vi "Begin.vi"() -> (0 "error out":errorcluster)   [LabVIEW 2023]
doc: "Called before other user functions, this VI is expected to open initial I/O refnums, load in file data, and do all program initialization. Notice that the <B>error out</B> terminal is simply used for data flow. Wiring it to other structures or subVIs ensures that this VI runs first."
uses:
  Robot Global Data.vi
  <vilib>/Rock Robotics/WPI/DriverStation/WPI_DriverStationRobotMode2.ctl
  <vilib>/Rock Robotics/WPI/Joystick/WPI_JoystickDeviceEnum.ctl
  <vilib>/Rock Robotics/WPI/ThirdParty/Phoenix-LabVIEW/Motor Controller/Controls/CTRE_Phoenix_MotorControl_FeedbackDevice_TalonFX.ctl
  <vilib>/Rock Robotics/WPI/ThirdParty/Phoenix-LabVIEW/Motor Controller/Controls/CTRE_Phoenix_MotorControl_NeutralMode.ctl
  <vilib>/Rock Robotics/WPI/ThirdParty/Phoenix-LabVIEW/Motor Controller/Controls/CTRE_Phoenix_MotorControl_TalonFXInvertType.ctl
  <vilib>/Rock Robotics/WPI/ThirdParty/Phoenix-LabVIEW/Motor Controller/Controls/CTRE_Phoenix_MotorControl_StatorCurrentLimitConfiguration.ctl
  <vilib>/Rock Robotics/WPI/ThirdParty/Phoenix-LabVIEW/CANCoder/Controls/CTRE_Phoenix_CANcoder_StatusFrame.ctl
  <vilib>/Rock Robotics/WPI/ThirdParty/REV Robotics/REVLib/Typedef/Spark MAX Idle Mode.ctl
  <vilib>/Rock Robotics/Network Tables/NT Write String Array.vi
  <vilib>/Rock Robotics/WPI/ThirdParty/Phoenix-LabVIEW/CANCoder/Controls/CTRE_Phoenix_CANcoder_SensorInitializationStrategy.ctl
  <vilib>/Rock Robotics/Network Tables/NT Write Number.vi
  <vilib>/Rock Robotics/Network Tables/NT Write String.vi
  <vilib>/Rock Robotics/WPI/ThirdParty/Phoenix-LabVIEW/CANdle/Controls/CTRE_Phoenix_CANdle_LEDStripType.ctl
  <vilib>/Rock Robotics/WPI/ThirdParty/Phoenix-LabVIEW/CANdle/Controls/CTRE_Phoenix_CANdle_Configurables.ctl
  <vilib>/Rock Robotics/SystemInterfaces/DIO/FPGA_DIOChannel.ctl
  <vilib>/Rock Robotics/Network Tables/NT Write Boolean.vi
  <vilib>/Rock Robotics/WPI/Switch/WPI_SwitchOpenLimit.vi
  <vilib>/Rock Robotics/WPI/ThirdParty/REV Robotics/REVLib/SubVI/Public/SPARK Open Brushless.vi
  <vilib>/Rock Robotics/WPI/ThirdParty/REV Robotics/REVLib/Typedef/Closed Loop Voltage Mode.ctl
  <vilib>/Rock Robotics/WPI/ThirdParty/REV Robotics/REVLib/Typedef/SPARK PID Gains.ctl
  <vilib>/Rock Robotics/WPI/ThirdParty/REV Robotics/REVLib/Typedef/SPARK Feedback Sensor.ctl
  <vilib>/Rock Robotics/WPI/ThirdParty/REV Robotics/REVLib/SubVI/Public/SPARK Configure Closed Loop Basic.vi
  <vilib>/Rock Robotics/WPI/ThirdParty/REV Robotics/REVLib/SubVI/Public/SPARK Configure Closed Loop MAXMotion.vi
  <vilib>/Rock Robotics/WPI/ThirdParty/REV Robotics/REVLib/SubVI/Public/SPARK Configure Basic Idle Mode.vi
  <vilib>/Rock Robotics/WPI/ThirdParty/REV Robotics/REVLib/SubVI/Public/SPARK Configure Power Smart Current Limit.vi
  <vilib>/Rock Robotics/WPI/ThirdParty/REV Robotics/REVLib/SubVI/Public/SPARK Configure Encoder Conversion Factors.vi
  <vilib>/Rock Robotics/WPI/ThirdParty/REV Robotics/REVLib/SubVI/Public/SPARK Configure Closed Loop Gains.vi
  <vilib>/Rock Robotics/WPI/ThirdParty/REV Robotics/REVLib/SubVI/Public/SPARK Configure Closed Loop Voltage Mode.vi
  <vilib>/Rock Robotics/Network Tables/NT Write Numeric Array.vi
  <vilib>/Rock Robotics/WPI/ThirdParty/REV Robotics/REVLib/SubVI/Public/SPARK Configure Soft Limit Reverse.vi
  <vilib>/Rock Robotics/WPI/ThirdParty/REV Robotics/REVLib/SubVI/Public/SPARK Configure Soft Limit Forward.vi
panel:
  in  "error in":errorcluster
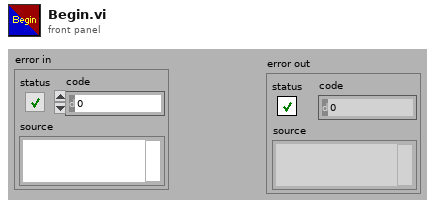
[diagram p1: front panel]
types:
  T1 = typedef "WPI_JoystickDeviceEnum.ctl" = enum16{"USB 0", "USB 1", "USB 2", "USB 3", "USB 4", "USB 5"}
  T2 = typedef "WPI_DriverStationRobotMode2.ctl" = enum16{"Autonomous Disabled", "Autonomous Enabled", "Teleop Disabled", "Teleop Enabled", "Disconnected", "Finish", "Test Disabled", "Test Enabled", "Emergency Stopped"}
  T3 = typedef "WPI_JoystickDevRef.ctl" = cluster{"Device":T1}
  T4 = typedef "CTRE_Phoenix_CANdle_Configurables.ctl" = cluster{"LED Strip Type":T5, "Brightness Scalar":dbl, "Disable LEDs when LoS":bool, "Status LED Off When Active":bool, "VBatOutputMode":u16}
  T5 = typedef "CTRE_Phoenix_CANdle_LEDStripType.ctl" = u16
  T6 = typedef "CTRE_Phoenix_CANdle_DeviceRef.ctl" = cluster{"DeviceStatus":errorcluster, "Device Number":u8, "Handle":u64, "UsageFrame":u32, "Library Path":path}
  T7 = typedef "SPARK Feedback Sensor.ctl" = enum16{"No Sensor", "Primary Encoder", "Analog Sensor", "Alternate or External Encoder", "Duty Cycle Sensor"}
  T8 = typedef "Spark MAX Idle Mode.ctl" = enum16{"Coast", "Brake"}
  T9 = typedef "SPARK PID Gains.ctl" = cluster{"kP":dbl, "kI":dbl, "kD":dbl}
  T10 = typedef "Closed Loop Voltage Mode.ctl" = enum16{"Disabled", "Voltage Output", "Voltage Compensation"}
  T11 = typedef "CTRE_Phoenix_MotorControl_StatorCurrentLimitConfiguration.ctl" = cluster{"Enable?":bool, "Current Limit":dbl, "Threshold Current":dbl, "Threshold Time":dbl}
  T12 = typedef "CTRE_Phoenix_MotorControl_NeutralMode.ctl" = enum8{"EEPROMSetting", "Override to Coast", "Override to Brake"}
  T13 = typedef "CTRE_Phoenix_MotorControl_TalonFXInvertType.ctl" = enum16{"Counter-Clockwise", "Clockwise"}
  T14 = typedef "FPGA_DIOChannel.ctl" = enum8{"DIO 0", "DIO 1", "DIO 2", "DIO 3", "DIO 4", "DIO 5", "DIO 6", "DIO 7", "DIO 8", "DIO 9", "DIO MXP 0", "DIO MXP 1", "DIO MXP 2", "DIO MXP 3", "DIO MXP 4", "DIO MXP 5", "DIO MXP 6", "DIO MXP 7", "DIO MXP 8", "DIO MXP 9", "DIO MXP 10", "DIO MXP 11", "DIO MXP 12", "DIO MXP 13", "DIO MXP 14", "DIO MXP 15", "SPI Port CS1", "SPI Port CS2", "SPI Port CS3", "SPI Port MISO", "SPI Port MOSI", "Invalid"}
  T15 = typedef "CTRE_Phoenix_CANcoder_SensorInitializationStrategy.ctl" = enum16{"Boot To Zero", "Boot To Absolute Position"}
  T16 = typedef "CTRE_Phoenix_MotorControl_FeedbackDevice_TalonFX.ctl" = i8
  T17 = typedef "CTRE_Phoenix_CANcoder_StatusFrame.ctl" = u32
  T18 = typedef "WPI_MotorControlDeviceRef.ctl" = cluster{"DeviceStatus":errorcluster, "Type":T19, "PWM":cluster{"PWM Channel":T20, "DeadBand":T21}, "CAN":cluster{"Device Number":u8, "SetOutput VI Ref":variant, "GetOutput VI Ref":variant, "Enable VI Ref":variant, "Disable VI Ref":variant, "Data":variant}, "Invert":bool, "DIO PWM":cluster{"PWM \"Enable\" Channel":T20, "DIOChannel":T14, "PWM Rate":dbl}}
  T19 = typedef "WPI_MotorControlType.ctl" = enum16{"PWM", "CAN", "DIO PWM"}
  T20 = typedef "FPGA_DIOPWMChannel.ctl" = enum8{"PWM 0", "PWM 1", "PWM 2", "PWM 3", "PWM 4", "PWM 5", "PWM 6", "PWM 7", "PWM 8", "PWM 9", "PWM MXP 0", "PWM MXP 1", "PWM MXP 2", "PWM MXP 3", "PWM MXP 4", "PWM MXP 5", "PWM MXP 6", "PWM MXP 7", "PWM MXP 8", "PWM MXP 9", "Invalid"}
  T21 = typedef "WPI_PWMDeadband.ctl" = cluster{"Name":string, "maxPositivePwm":i32, "minPositivePwm":i32, "centerPwm":i32, "maxNegativePwm":i32, "minNegativePwm":i32, "angularRange":u16}
  T22 = typedef "WPI_SwitchDevRef.ctl" = cluster{"DevStatus":errorcluster, "DIO Channel":T14, "CntIndex":T23, "Normally Closed":bool}
  T23 = typedef "FPGA_CounterCtrSystemIndex.ctl" = enum8{"Ctr 0", "Ctr 1", "Ctr 2", "Ctr 3", "Ctr 4", "Ctr 5", "Ctr 6", "Ctr 7", "Invalid"}
  T24 = typedef "CTRE_Phoenix_CANcoder_DeviceRef.ctl" = cluster{"DeviceStatus":errorcluster, "Device Number":u8, "Handle":u64, "UsageFrame":u32, "Library Path":path}
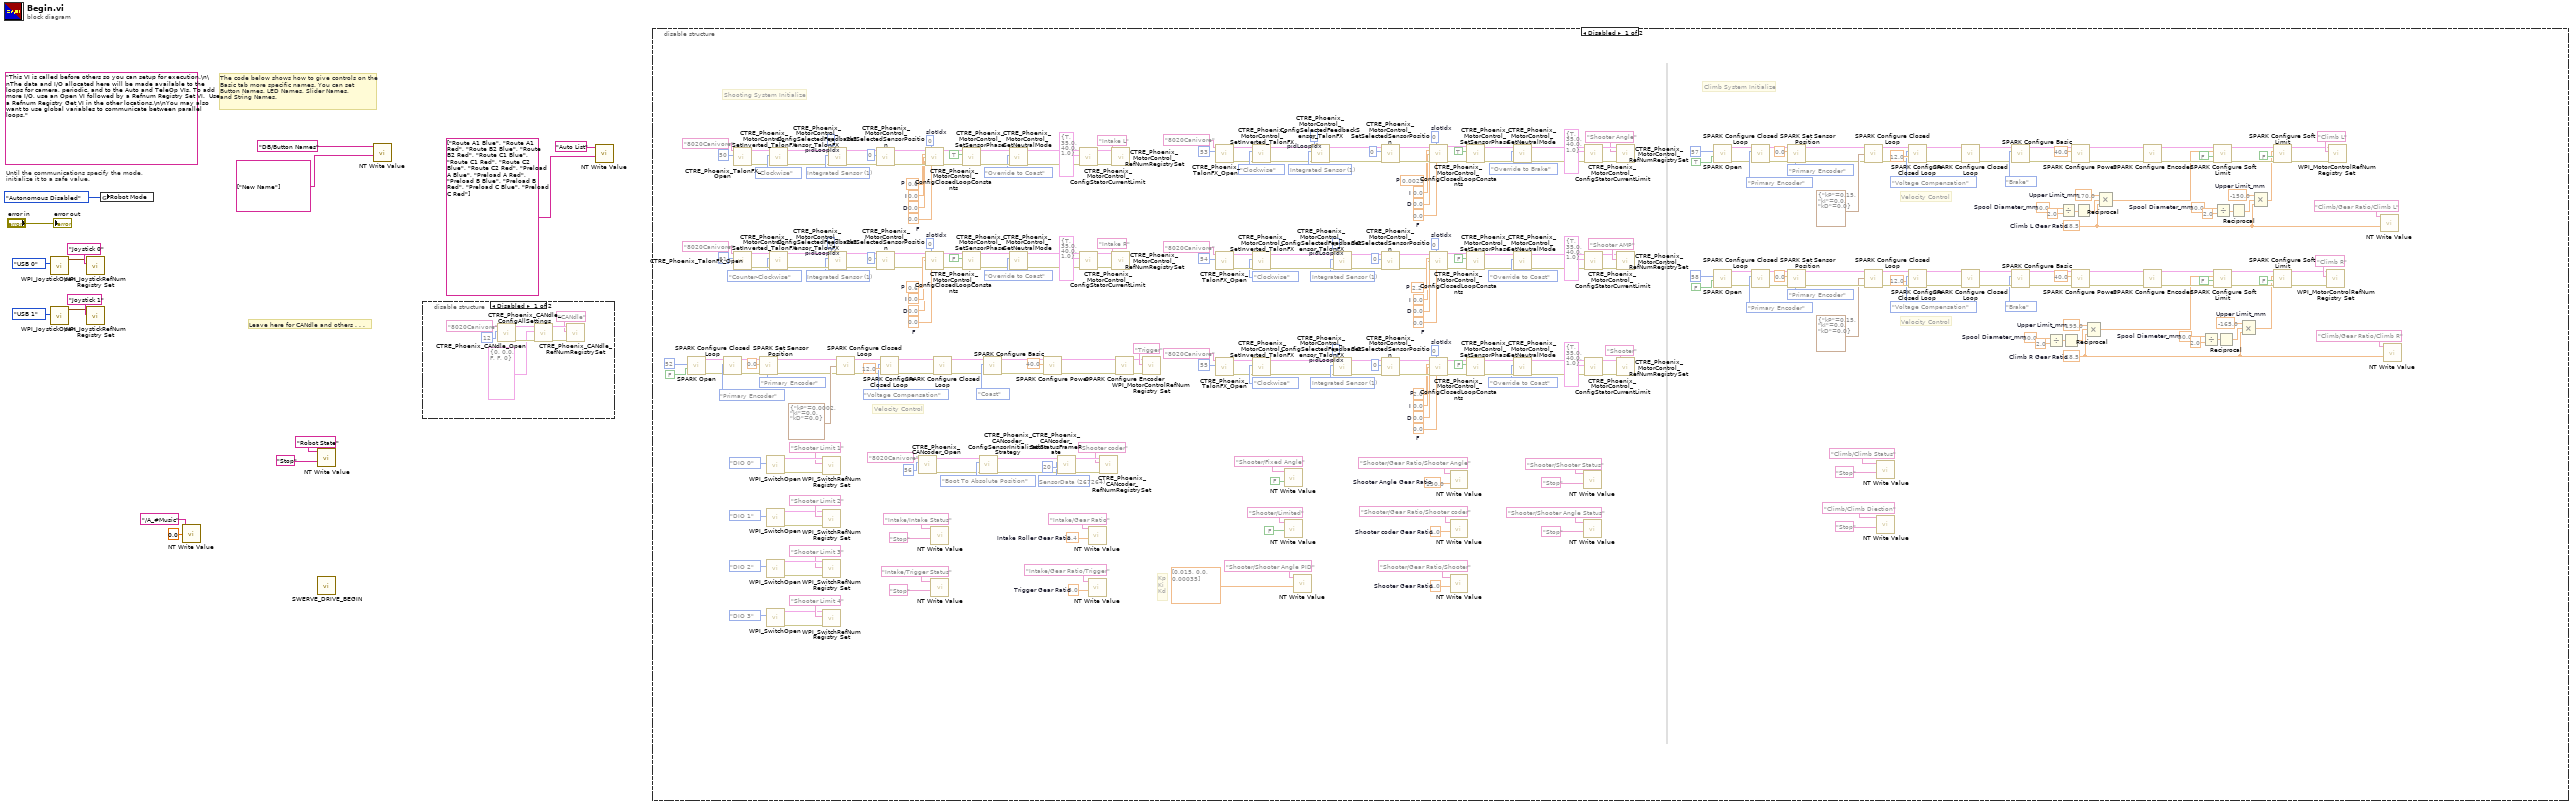
[diagram p0: block diagram]
diagram:
  (unwired) "This VI is called before others so you can setup for execution.\n\nThe data and I/O allocated here will be made available to the loops for camera, periodic, and to the Auto and TeleOp VIs. To add more I/O, use an Open VI followed by a Refnum Registry Set VI.  Use a Refnum Registry Get VI in the other locations.\n\nYou may also want to use global variables to communicate between parallel loops."
  # "Leave here for CANdle and others . . ."
  # "The code below shows how to give controls on the\nBasic tab more specific names. You can set\nButton Names, LED Names, Slider Names,\nand String Names."
  # "Until the communications specify the mode,\ninitialize it to a safe value."
  n1 = call <vilib>:"WPI_JoystickOpen.vi"("JoystickDevice"=WPI_JoystickDeviceEnum."USB 0") -> ("JoystickDevRef"=w14:T3)  [unwired: 10 in]
  n2 = call <vilib>:"WPI_JoystickOpen.vi"("JoystickDevice"=WPI_JoystickDeviceEnum."USB 1") -> ("JoystickDevRef"=w8:T3)  [unwired: 10 in]
  n3 = call <vilib>:"WPI_JoystickRefNum Registry Set.vi"("refnum name"="Joystick 0", "JoystickDevRef"=w14) -> ()  [unwired: 8 in, 2 out]
  n4 = call <vilib>:"WPI_JoystickRefNum Registry Set.vi"("refnum name"="Joystick 1", "JoystickDevRef"=w8) -> ()  [unwired: 8 in, 2 out]
  n5 = global write "Robot Global Data.vi" "Robot Mode"(WPI_DriverStationRobotMode2."Autonomous Disabled" ("Robot Mode")) -> ()
  n6 = call-poly <vilib>:"NT Write Value.vi"("value"=0.0, "name"="/A_#Music") -> ()  [unwired: 9 in, 1 out]
  n7 = call-poly <vilib>:"NT Write Value.vi"("value"="Stop" ("default value"), "name"="Robot State") -> ()  [unwired: 9 in, 1 out]
  n8 = call "SWERVE_DRIVE_BEGIN.vi"() -> ()  [unwired: 11 in, 1 out]
  n9 = call-poly <vilib>:"NT Write Value.vi"("value"=string[] ["New Name"], "name"="DB/Button Names" ("Name")) -> ()  [unwired: 9 in, 1 out]
  n10 = disable-structure shown="Disabled" {
    frame Disabled {
      n11 = call <vilib>:"CTRE_Phoenix_CANdle_Open.vi"("Device Number"=u8 12, "CAN Bus"="8020Canivore") -> ("error out"=w24:errorcluster, "CTRE_CANdle_DeviceRef"=w23:T6)  [unwired: 8 in]
      n12 = call <vilib>:"CTRE_Phoenix_CANdle_ConfigAllSettings.vi"("error in (no error)"=w24, "CANdle Configurables"=T4 {"LED Strip Type"=0, "Brightness Scalar"=0.0, "Disable LEDs when LoS"=FALSE, "Status LED Off When Active"=FALSE, "VBatOutputMode"=0}, "CTRE_CANdle_DeviceRef"=w23) -> ("error out"=w21:errorcluster, "CTRE_CANdle_DeviceRef"=w20:T6)  [unwired: 7 in]
      n13 = call <vilib>:"CTRE_Phoenix_CANdle_RefNumRegistrySet.vi"("error in (no error)"=w21, "refnum name"="CANdle", "CTRE_CANdle_DeviceRef"=w20) -> ()  [unwired: 7 in, 2 out]
    }
    frame Enabled {
    }
  }
  n14 = call-poly <vilib>:"NT Write Value.vi"("value"=string[] ["Route A1 Blue", "Route A1 Red", "Route B2 Blue", "Route B2 Red", "Route C1 Blue", "Route C1 Red", "Route C2 Blue", "Route C2 Red", "Preload A Blue", "Preload A Red", "Preload B Blue", "Preload B Red", "Preload C Blue", "Preload C Red"] ("String Array"), "name"="Auto List" ("Name")) -> ()  [unwired: 9 in, 1 out]
  n15 = disable-structure shown="Disabled" {
    frame Disabled {
      w124 = -165.0  # Upper Limit_mm
      w120 = 30.0  # Spool Diameter_mm
      w126 = -150.0  # Upper Limit_mm
      w130 = 30.0  # Spool Diameter_mm
      w149 = 0  # slotIdx
      w148 = 0.0  # F
      w152 = 0.0  # D
      w151 = 0.0  # I
      w150 = 0.6  # P
      w143 = 0  # pidLoopIdx
      w139 = T16 1 items=["Integrated Sensor"=1, "Sensor Sum (S0 + S1)"=9, "Sensor Difference (D0 - D1)"=10, "Remote Source 0"=11, "Remote Source 1"=12, "None"=14, "Software Emulated"=15] ("Talon FX Feedback Device")
      w181 = 0  # slotIdx
      w182 = 0.0  # F
      w178 = 0.0  # D
      w179 = 0.0  # I
      w180 = 0.6  # P
      w187 = 0  # pidLoopIdx
      w191 = T16 1 items=["Integrated Sensor"=1, "Sensor Sum (S0 + S1)"=9, "Sensor Difference (D0 - D1)"=10, "Remote Source 0"=11, "Remote Source 1"=12, "None"=14, "Software Emulated"=15] ("Talon FX Feedback Device")
      w214 = 0  # slotIdx
      w213 = 0.0  # F
      w217 = 0.0  # D
      w216 = 0.0  # I
      w215 = 2.0  # P
      w208 = 0  # pidLoopIdx
      w204 = T16 1 items=["Integrated Sensor"=1, "Sensor Sum (S0 + S1)"=9, "Sensor Difference (D0 - D1)"=10, "Remote Source 0"=11, "Remote Source 1"=12, "None"=14, "Software Emulated"=15] ("Talon FX Feedback Device")
      w243 = 0  # slotIdx
      w244 = 0.0  # F
      w240 = 0.0  # D
      w241 = 0.0  # I
      w242 = 2.2  # P
      w249 = 0  # pidLoopIdx
      w253 = T16 1 items=["Integrated Sensor"=1, "Sensor Sum (S0 + S1)"=9, "Sensor Difference (D0 - D1)"=10, "Remote Source 0"=11, "Remote Source 1"=12, "None"=14, "Software Emulated"=15] ("Talon FX Feedback Device")
      w279 = 5.0  # Trigger Gear Ratio
      w277 = 2.4  # Intake Roller Gear Ratio
      w281 = 150.0  # Shooter Angle Gear Ratio
      w283 = 1.0  # Shooter coder Gear Ratio
      w296 = 170.0  # Upper Limit_mm
      w292 = 30.0  # Spool Diameter_mm
      w125 = 28.5  # Climb L Gear Ratio
      w297 = 195.0  # Upper Limit_mm
      w301 = 30.0  # Spool Diameter_mm
      w119 = 28.5  # Climb R Gear Ratio
      w314 = 1.0  # Shooter Gear Ratio
      w323 = T17 267264 items=["SensorData"=267264, "VbatAndFaults"=267328] ("CANcoder Status Frame")
      w349 = 0  # slotIdx
      w348 = 0.0  # F
      w352 = 0.0  # D
      w351 = 0.0  # I
      w350 = 0.0025  # P
      w344 = 0  # pidLoopIdx
      w340 = T16 1 items=["Integrated Sensor"=1, "Sensor Sum (S0 + S1)"=9, "Sensor Difference (D0 - D1)"=10, "Remote Source 0"=11, "Remote Source 1"=12, "None"=14, "Software Emulated"=15] ("Talon FX Feedback Device")
      # "Velocity Control"
      # "Velocity Control"
      # "Velocity Control"
      # "Kp\nKi\nKd"
      # "Climb System Initialize"
      # "Shooting System Initialize"
      n16 = call-poly <vilib>:"SPARK Open.vi"("Invert"=FALSE, "Device Number"=u8 52) -> ("error out"=w95:errorcluster, "MotorControlDeviceRef"=w96:T18)  [unwired: 8 in]
      n17 = call-poly <vilib>:"SPARK Configure Closed Loop.vi"("error in"=w95, "Feedback Sensor (Primary Encoder)"=SPARK_Feedback_Sensor."Primary Encoder", "MotorControlDeviceRef in"=w96) -> ("error out"=w100:errorcluster, "MotorControlDeviceRef out"=w102:T18)  [unwired: 7 in]
      n18 = call <vilib>:"CTRE_Phoenix_TalonFX_Open.vi"("Device Number"=u8 50, "CAN Bus"="8020Canivore") -> ("error out"=w133:errorcluster, "PhoenixMotorControlDevRef"=w134:T18)  [unwired: 8 in]
      n19 = call <vilib>:"CTRE_Phoenix_TalonFX_Open.vi"("Device Number"=u8 51, "CAN Bus"="8020Canivore") -> ("error out"=w197:errorcluster, "PhoenixMotorControlDevRef"=w196:T18)  [unwired: 8 in]
      n20 = call <vilib>:"SPARK Set Sensor Position.vi"("Sensor (Primary Encoder)"=enum16{"Primary Encoder", "Alt/Ext Encoder"}."Primary Encoder", "error in"=w100, "Position"=0.0, "MotorControlDeviceRef"=w102) -> ("error out"=w98:errorcluster, "MotorControlDeviceRef"=w99:T18)  [unwired: 6 in]
      n21 = call-poly <vilib>:"WPI_SwitchOpen.vi"("DIO Channel"=FPGA_DIOChannel."DIO 0") -> ("error out"=w291:errorcluster, "SwitchDevRef"=w290:T22)  [unwired: 9 in]
      n22 = call-poly <vilib>:"WPI_SwitchOpen.vi"("DIO Channel"=FPGA_DIOChannel."DIO 1") -> ("error out"=w271:errorcluster, "SwitchDevRef"=w272:T22)  [unwired: 9 in]
      n23 = call-poly <vilib>:"WPI_SwitchOpen.vi"("DIO Channel"=FPGA_DIOChannel."DIO 2") -> ("error out"=w270:errorcluster, "SwitchDevRef"=w269:T22)  [unwired: 9 in]
      n24 = call-poly <vilib>:"WPI_SwitchOpen.vi"("DIO Channel"=FPGA_DIOChannel."DIO 3") -> ("error out"=w263:errorcluster, "SwitchDevRef"=w264:T22)  [unwired: 9 in]
      n25 = call <vilib>:"CTRE_Phoenix_MotorControl_SetInverted_TalonFX.vi"("error in (no error)"=w133, "Invert Type"=CTRE_Phoenix_MotorControl_TalonFXInvertType."Clockwise", "PhoenixMotorControlDevRef"=w134) -> ("error out"=w137:errorcluster, "PhoenixMotorControlDevRef"=w138:T18)  [unwired: 7 in]
      n26 = call <vilib>:"CTRE_Phoenix_MotorControl_SetInverted_TalonFX.vi"("error in (no error)"=w197, "Invert Type"=CTRE_Phoenix_MotorControl_TalonFXInvertType."Counter-Clockwise", "PhoenixMotorControlDevRef"=w196) -> ("error out"=w193:errorcluster, "PhoenixMotorControlDevRef"=w192:T18)  [unwired: 7 in]
      n27 = call <vilib>:"WPI_SwitchRefNum Registry Set.vi"("error in (no error)"=w291, "refnum name"="Shooter Limit 1", "SwitchDevRef"=w290) -> ()  [unwired: 7 in, 2 out]
      n28 = call <vilib>:"WPI_SwitchRefNum Registry Set.vi"("error in (no error)"=w271, "refnum name"="Shooter Limit 2", "SwitchDevRef"=w272) -> ()  [unwired: 7 in, 2 out]
      n29 = call <vilib>:"WPI_SwitchRefNum Registry Set.vi"("error in (no error)"=w270, "refnum name"="Shooter Limit 3", "SwitchDevRef"=w269) -> ()  [unwired: 7 in, 2 out]
      n30 = call <vilib>:"WPI_SwitchRefNum Registry Set.vi"("error in (no error)"=w263, "refnum name"="Shooter Limit 4", "SwitchDevRef"=w264) -> ()  [unwired: 7 in, 2 out]
      n31 = call <vilib>:"CTRE_Phoenix_MotorControl_ConfigSelectedFeedbackSensor_TalonFX.vi"("error in (no error)"=w137, "pidLoopIdx"=w143, "Talon FX Feedback Device"=w139, "PhoenixMotorControlDevRef"=w138) -> ("error out"=w147:errorcluster, "PhoenixMotorControlDevRef"=w146:T18)  [unwired: 6 in]
      n32 = call <vilib>:"CTRE_Phoenix_MotorControl_ConfigSelectedFeedbackSensor_TalonFX.vi"("error in (no error)"=w193, "pidLoopIdx"=w187, "Talon FX Feedback Device"=w191, "PhoenixMotorControlDevRef"=w192) -> ("error out"=w183:errorcluster, "PhoenixMotorControlDevRef"=w184:T18)  [unwired: 6 in]
      n33 = call-poly <vilib>:"SPARK Configure Closed Loop.vi"("error in"=w98, "PID Gains"=T9 {"kP"=0.0002, "kI"=0.0, "kD"=0.0}, "MotorControlDeviceRef in"=w99) -> ("error out"=w114:errorcluster, "MotorControlDeviceRef out"=w115:T18)  [unwired: 7 in]
      n34 = call <vilib>:"CTRE_Phoenix_MotorControl_SetSelectedSensorPosition.vi"("error in (no error)"=w147, "New Sensor Position"=0, "PhoenixMotorControlDevRef"=w146) -> ("error out"=w154:errorcluster, "PhoenixMotorControlDevRef"=w153:T18)  [unwired: 7 in]
      n35 = call <vilib>:"CTRE_Phoenix_MotorControl_SetSelectedSensorPosition.vi"("error in (no error)"=w183, "New Sensor Position"=0, "PhoenixMotorControlDevRef"=w184) -> ("error out"=w176:errorcluster, "PhoenixMotorControlDevRef"=w177:T18)  [unwired: 7 in]
      n36 = call-poly <vilib>:"SPARK Configure Closed Loop.vi"("error in (no error)"=w114, "Compensated Nominal Voltage"=12.0, "Voltage Mode (Disabled)"=Closed_Loop_Voltage_Mode."Voltage Compensation", "MotorControlDeviceRef in"=w115) -> ("error out"=w106:errorcluster, "MotorControlDeviceRef out"=w107:T18)  [unwired: 6 in]
      n37 = call <vilib>:"CTRE_Phoenix_CANcoder_Open.vi"("Device Number"=56, "CAN Bus"="8020Canivore") -> ("error out"=w317:errorcluster, "CTRE_CANcoder_DeviceRef"=w319:T24)  [unwired: 8 in]
      n38 = call <vilib>:"CTRE_Phoenix_MotorControl_ConfigClosedLoopConstants.vi"("PhoenixMotorControlDevRef"=w153, "slotIdx"=w149, "P"=w150, "I"=w151, "D"=w152, "error in (no error)"=w154, "F"=w148) -> ("PhoenixMotorControlDevRef"=w155:T18, "error out"=w156:errorcluster)  [unwired: 7 in]
      n39 = call <vilib>:"CTRE_Phoenix_MotorControl_ConfigClosedLoopConstants.vi"("PhoenixMotorControlDevRef"=w177, "slotIdx"=w181, "P"=w180, "I"=w179, "D"=w178, "error in (no error)"=w176, "F"=w182) -> ("PhoenixMotorControlDevRef"=w175:T18, "error out"=w174:errorcluster)  [unwired: 7 in]
      n40 = call-poly <vilib>:"NT Write Value.vi"("value"="Stop" ("default value"), "name"="Intake/Intake Status") -> ()  [unwired: 9 in, 1 out]
      n41 = call-poly <vilib>:"NT Write Value.vi"("value"="Stop" ("default value"), "name"="Intake/Trigger Status") -> ()  [unwired: 9 in, 1 out]
      n42 = call-poly <vilib>:"SPARK Configure Closed Loop.vi"("error in (no error)"=w106, "MotorControlDeviceRef in"=w107) -> ("error out"=w104:errorcluster, "MotorControlDeviceRef out"=w105:T18)  [unwired: 8 in]
      n43 = call <vilib>:"CTRE_Phoenix_MotorControl_SetSensorPhase.vi"("error in (no error)"=w156, "PhaseSensor"=TRUE, "PhoenixMotorControlDevRef"=w155) -> ("error out"=w158:errorcluster, "PhoenixMotorControlDevRef"=w157:T18)  [unwired: 7 in]
      n44 = call <vilib>:"CTRE_Phoenix_MotorControl_SetSensorPhase.vi"("error in (no error)"=w174, "PhaseSensor"=FALSE, "PhoenixMotorControlDevRef"=w175) -> ("error out"=w172:errorcluster, "PhoenixMotorControlDevRef"=w173:T18)  [unwired: 7 in]
      n45 = call <vilib>:"CTRE_Phoenix_CANcoder_ConfigSensorInitializationStrategy.vi"("error in"=w317, "Sensor Initialization Strategy"=CTRE_Phoenix_CANcoder_SensorInitializationStrategy."Boot To Absolute Position", "CTRE_CANcoder_DeviceRef"=w319) -> ("error out"=w316:errorcluster, "CTRE_CANcoder_DeviceRef"=w318:T24)  [unwired: 7 in]
      n46 = call-poly <vilib>:"SPARK Configure Basic.vi"("error in (no error)"=w104, "Idle Mode"=Spark_MAX_Idle_Mode."Coast", "MotorControlDeviceRef in"=w105) -> ("error out"=w108:errorcluster, "MotorControlDeviceRef out"=w109:T18)  [unwired: 7 in]
      n47 = call <vilib>:"CTRE_Phoenix_MotorControl_SetNeutralMode.vi"("error in (no error)"=w158, "Motor Control Neutral Mode"=CTRE_Phoenix_MotorControl_NeutralMode."Override to Coast", "PhoenixMotorControlDevRef"=w157) -> ("error out"=w162:errorcluster, "PhoenixMotorControlDevRef"=w161:T18)  [unwired: 7 in]
      n48 = call <vilib>:"CTRE_Phoenix_MotorControl_SetNeutralMode.vi"("error in (no error)"=w172, "Motor Control Neutral Mode"=CTRE_Phoenix_MotorControl_NeutralMode."Override to Coast", "PhoenixMotorControlDevRef"=w173) -> ("error out"=w168:errorcluster, "PhoenixMotorControlDevRef"=w169:T18)  [unwired: 7 in]
      n49 = call-poly <vilib>:"SPARK Configure Power.vi"("error in (no error)"=w108, "Primay Current Limit (80A)"=40.0, "MotorControlDeviceRef in"=w109) -> ("error out"=w111:errorcluster, "MotorControlDeviceRef out"=w112:T18)  [unwired: 7 in]
      n50 = call <vilib>:"CTRE_Phoenix_CANcoder_SetStatusFrameRate.vi"("error in (no error)"=w316, "Period (ms)"=u8 20, "CANcoder Status Frame"=w323, "CTRE_CANcoder_DeviceRef"=w318) -> ("error out"=w326:errorcluster, "CTRE_CANcoder_DeviceRef"=w325:T24)  [unwired: 6 in]
      n51 = call <vilib>:"CTRE_Phoenix_MotorControl_ConfigStatorCurrentLimit.vi"("error in (no error)"=w162, "Stator Current Limit Configuration"=T11 {"Enable?"=TRUE, "Current Limit"=35.0, "Threshold Current"=40.0, "Threshold Time"=1.0}, "PhoenixMotorControlDevRef"=w161) -> ("error out"=w160:errorcluster, "PhoenixMotorControlDevRef"=w159:T18)  [unwired: 7 in]
      n52 = call <vilib>:"CTRE_Phoenix_MotorControl_ConfigStatorCurrentLimit.vi"("error in (no error)"=w168, "Stator Current Limit Configuration"=T11 {"Enable?"=TRUE, "Current Limit"=35.0, "Threshold Current"=40.0, "Threshold Time"=1.0}, "PhoenixMotorControlDevRef"=w169) -> ("error out"=w170:errorcluster, "PhoenixMotorControlDevRef"=w171:T18)  [unwired: 7 in]
      n53 = call-poly <vilib>:"NT Write Value.vi"("value"=w277, "name"="Intake/Gear Ratio") -> ()  [unwired: 9 in, 1 out]
      n54 = call-poly <vilib>:"NT Write Value.vi"("value"=w279, "name"="Intake/Gear Ratio/Trigger") -> ()  [unwired: 9 in, 1 out]
      n55 = call <vilib>:"CTRE_Phoenix_CANcoder_RefNumRegistrySet.vi"("error in (no error)"=w326, "refnum name"="Shooter coder", "CTRE_CANcoder_DeviceRef"=w325) -> ()  [unwired: 7 in, 2 out]
      n56 = call <vilib>:"CTRE_Phoenix_MotorControl_RefNumRegistrySet.vi"("error in (no error)"=w160, "refnum name"="Intake L", "PhoenixMotorControlDevRef"=w159) -> ()  [unwired: 7 in, 2 out]
      n57 = call <vilib>:"CTRE_Phoenix_MotorControl_RefNumRegistrySet.vi"("error in (no error)"=w170, "refnum name"="Intake R", "PhoenixMotorControlDevRef"=w171) -> ()  [unwired: 7 in, 2 out]
      n58 = call-poly <vilib>:"SPARK Configure Encoder.vi"("error in"=w111, "MotorControlDeviceRef in"=w112) -> ("error out"=w93:errorcluster, "MotorControlDeviceRef out"=w94:T18)  [unwired: 8 in]
      n59 = call <vilib>:"WPI_MotorControlRefNum Registry Set.vi"("error in (no error)"=w93, "refnum name"="Trigger", "MotorControlDevRef"=w94) -> ()  [unwired: 7 in, 2 out]
      n60 = call <vilib>:"CTRE_Phoenix_TalonFX_Open.vi"("Device Number"=u8 53, "CAN Bus"="8020Canivore") -> ("error out"=w334:errorcluster, "PhoenixMotorControlDevRef"=w335:T18)  [unwired: 8 in]
      n61 = call <vilib>:"CTRE_Phoenix_TalonFX_Open.vi"("Device Number"=u8 54, "CAN Bus"="8020Canivore") -> ("error out"=w259:errorcluster, "PhoenixMotorControlDevRef"=w258:T18)  [unwired: 8 in]
      n62 = call <vilib>:"CTRE_Phoenix_TalonFX_Open.vi"("Device Number"=u8 55, "CAN Bus"="8020Canivore") -> ("error out"=w198:errorcluster, "PhoenixMotorControlDevRef"=w199:T18)  [unwired: 8 in]
      n63 = call <vilib>:"CTRE_Phoenix_MotorControl_SetInverted_TalonFX.vi"("error in (no error)"=w334, "Invert Type"=CTRE_Phoenix_MotorControl_TalonFXInvertType."Clockwise", "PhoenixMotorControlDevRef"=w335) -> ("error out"=w338:errorcluster, "PhoenixMotorControlDevRef"=w339:T18)  [unwired: 7 in]
      n64 = call <vilib>:"CTRE_Phoenix_MotorControl_SetInverted_TalonFX.vi"("error in (no error)"=w259, "Invert Type"=CTRE_Phoenix_MotorControl_TalonFXInvertType."Clockwise", "PhoenixMotorControlDevRef"=w258) -> ("error out"=w255:errorcluster, "PhoenixMotorControlDevRef"=w254:T18)  [unwired: 7 in]
      n65 = call <vilib>:"CTRE_Phoenix_MotorControl_SetInverted_TalonFX.vi"("error in (no error)"=w198, "Invert Type"=CTRE_Phoenix_MotorControl_TalonFXInvertType."Clockwise", "PhoenixMotorControlDevRef"=w199) -> ("error out"=w202:errorcluster, "PhoenixMotorControlDevRef"=w203:T18)  [unwired: 7 in]
      n66 = call-poly <vilib>:"NT Write Value.vi"("value"=FALSE ("default value"), "name"="Shooter/Fixed Angle") -> ()  [unwired: 9 in, 1 out]
      n67 = call-poly <vilib>:"NT Write Value.vi"("value"=FALSE, "name"="Shooter/Limited") -> ()  [unwired: 9 in, 1 out]
      n68 = call-poly <vilib>:"NT Write Value.vi"("value"=dbl[] [0.015, 0.0, 0.00035], "name"="Shooter/Shooter Angle PID") -> ()  [unwired: 9 in, 1 out]
      n69 = call <vilib>:"CTRE_Phoenix_MotorControl_ConfigSelectedFeedbackSensor_TalonFX.vi"("error in (no error)"=w338, "pidLoopIdx"=w344, "Talon FX Feedback Device"=w340, "PhoenixMotorControlDevRef"=w339) -> ("error out"=w347:errorcluster, "PhoenixMotorControlDevRef"=w346:T18)  [unwired: 6 in]
      n70 = call <vilib>:"CTRE_Phoenix_MotorControl_ConfigSelectedFeedbackSensor_TalonFX.vi"("error in (no error)"=w255, "pidLoopIdx"=w249, "Talon FX Feedback Device"=w253, "PhoenixMotorControlDevRef"=w254) -> ("error out"=w245:errorcluster, "PhoenixMotorControlDevRef"=w246:T18)  [unwired: 6 in]
      n71 = call <vilib>:"CTRE_Phoenix_MotorControl_ConfigSelectedFeedbackSensor_TalonFX.vi"("error in (no error)"=w202, "pidLoopIdx"=w208, "Talon FX Feedback Device"=w204, "PhoenixMotorControlDevRef"=w203) -> ("error out"=w212:errorcluster, "PhoenixMotorControlDevRef"=w211:T18)  [unwired: 6 in]
      n72 = call <vilib>:"CTRE_Phoenix_MotorControl_SetSelectedSensorPosition.vi"("error in (no error)"=w347, "New Sensor Position"=0, "PhoenixMotorControlDevRef"=w346) -> ("error out"=w354:errorcluster, "PhoenixMotorControlDevRef"=w353:T18)  [unwired: 7 in]
      n73 = call <vilib>:"CTRE_Phoenix_MotorControl_SetSelectedSensorPosition.vi"("error in (no error)"=w245, "New Sensor Position"=0, "PhoenixMotorControlDevRef"=w246) -> ("error out"=w238:errorcluster, "PhoenixMotorControlDevRef"=w239:T18)  [unwired: 7 in]
      n74 = call <vilib>:"CTRE_Phoenix_MotorControl_SetSelectedSensorPosition.vi"("error in (no error)"=w212, "New Sensor Position"=0, "PhoenixMotorControlDevRef"=w211) -> ("error out"=w219:errorcluster, "PhoenixMotorControlDevRef"=w218:T18)  [unwired: 7 in]
      n75 = call <vilib>:"CTRE_Phoenix_MotorControl_ConfigClosedLoopConstants.vi"("PhoenixMotorControlDevRef"=w353, "slotIdx"=w349, "P"=w350, "I"=w351, "D"=w352, "error in (no error)"=w354, "F"=w348) -> ("PhoenixMotorControlDevRef"=w355:T18, "error out"=w356:errorcluster)  [unwired: 7 in]
      n76 = call <vilib>:"CTRE_Phoenix_MotorControl_ConfigClosedLoopConstants.vi"("PhoenixMotorControlDevRef"=w239, "slotIdx"=w243, "P"=w242, "I"=w241, "D"=w240, "error in (no error)"=w238, "F"=w244) -> ("PhoenixMotorControlDevRef"=w237:T18, "error out"=w236:errorcluster)  [unwired: 7 in]
      n77 = call <vilib>:"CTRE_Phoenix_MotorControl_ConfigClosedLoopConstants.vi"("PhoenixMotorControlDevRef"=w218, "slotIdx"=w214, "P"=w215, "I"=w216, "D"=w217, "error in (no error)"=w219, "F"=w213) -> ("PhoenixMotorControlDevRef"=w220:T18, "error out"=w221:errorcluster)  [unwired: 7 in]
      n78 = call-poly <vilib>:"NT Write Value.vi"("value"=w281, "name"="Shooter/Gear Ratio/Shooter Angle") -> ()  [unwired: 9 in, 1 out]
      n79 = call-poly <vilib>:"NT Write Value.vi"("value"=w283, "name"="Shooter/Gear Ratio/Shooter coder") -> ()  [unwired: 9 in, 1 out]
      n80 = call-poly <vilib>:"NT Write Value.vi"("value"=w314, "name"="Shooter/Gear Ratio/Shooter") -> ()  [unwired: 9 in, 1 out]
      n81 = call <vilib>:"CTRE_Phoenix_MotorControl_SetSensorPhase.vi"("error in (no error)"=w356, "PhaseSensor"=TRUE, "PhoenixMotorControlDevRef"=w355) -> ("error out"=w358:errorcluster, "PhoenixMotorControlDevRef"=w357:T18)  [unwired: 7 in]
      n82 = call <vilib>:"CTRE_Phoenix_MotorControl_SetSensorPhase.vi"("error in (no error)"=w236, "PhaseSensor"=FALSE, "PhoenixMotorControlDevRef"=w237) -> ("error out"=w234:errorcluster, "PhoenixMotorControlDevRef"=w235:T18)  [unwired: 7 in]
      n83 = call <vilib>:"CTRE_Phoenix_MotorControl_SetSensorPhase.vi"("error in (no error)"=w221, "PhaseSensor"=FALSE, "PhoenixMotorControlDevRef"=w220) -> ("error out"=w223:errorcluster, "PhoenixMotorControlDevRef"=w222:T18)  [unwired: 7 in]
      n84 = call <vilib>:"CTRE_Phoenix_MotorControl_SetNeutralMode.vi"("error in (no error)"=w358, "Motor Control Neutral Mode"=CTRE_Phoenix_MotorControl_NeutralMode."Override to Brake", "PhoenixMotorControlDevRef"=w357) -> ("error out"=w362:errorcluster, "PhoenixMotorControlDevRef"=w361:T18)  [unwired: 7 in]
      n85 = call <vilib>:"CTRE_Phoenix_MotorControl_SetNeutralMode.vi"("error in (no error)"=w234, "Motor Control Neutral Mode"=CTRE_Phoenix_MotorControl_NeutralMode."Override to Coast", "PhoenixMotorControlDevRef"=w235) -> ("error out"=w230:errorcluster, "PhoenixMotorControlDevRef"=w231:T18)  [unwired: 7 in]
      n86 = call <vilib>:"CTRE_Phoenix_MotorControl_SetNeutralMode.vi"("error in (no error)"=w223, "Motor Control Neutral Mode"=CTRE_Phoenix_MotorControl_NeutralMode."Override to Coast", "PhoenixMotorControlDevRef"=w222) -> ("error out"=w227:errorcluster, "PhoenixMotorControlDevRef"=w226:T18)  [unwired: 7 in]
      n87 = call-poly <vilib>:"NT Write Value.vi"("value"="Stop" ("default value"), "name"="Shooter/Shooter Status") -> ()  [unwired: 9 in, 1 out]
      n88 = call-poly <vilib>:"NT Write Value.vi"("value"="Stop" ("default value"), "name"="Shooter/Shooter Angle Status") -> ()  [unwired: 9 in, 1 out]
      n89 = call <vilib>:"CTRE_Phoenix_MotorControl_ConfigStatorCurrentLimit.vi"("error in (no error)"=w362, "Stator Current Limit Configuration"=T11 {"Enable?"=TRUE, "Current Limit"=35.0, "Threshold Current"=40.0, "Threshold Time"=1.0}, "PhoenixMotorControlDevRef"=w361) -> ("error out"=w360:errorcluster, "PhoenixMotorControlDevRef"=w359:T18)  [unwired: 7 in]
      n90 = call <vilib>:"CTRE_Phoenix_MotorControl_ConfigStatorCurrentLimit.vi"("error in (no error)"=w230, "Stator Current Limit Configuration"=T11 {"Enable?"=TRUE, "Current Limit"=35.0, "Threshold Current"=40.0, "Threshold Time"=1.0}, "PhoenixMotorControlDevRef"=w231) -> ("error out"=w232:errorcluster, "PhoenixMotorControlDevRef"=w233:T18)  [unwired: 7 in]
      n91 = call <vilib>:"CTRE_Phoenix_MotorControl_ConfigStatorCurrentLimit.vi"("error in (no error)"=w227, "Stator Current Limit Configuration"=T11 {"Enable?"=TRUE, "Current Limit"=35.0, "Threshold Current"=40.0, "Threshold Time"=1.0}, "PhoenixMotorControlDevRef"=w226) -> ("error out"=w225:errorcluster, "PhoenixMotorControlDevRef"=w224:T18)  [unwired: 7 in]
      n92 = call <vilib>:"CTRE_Phoenix_MotorControl_RefNumRegistrySet.vi"("error in (no error)"=w360, "refnum name"="Shooter Angle", "PhoenixMotorControlDevRef"=w359) -> ()  [unwired: 7 in, 2 out]
      n93 = call <vilib>:"CTRE_Phoenix_MotorControl_RefNumRegistrySet.vi"("error in (no error)"=w232, "refnum name"="Shooter AMP", "PhoenixMotorControlDevRef"=w233) -> ()  [unwired: 7 in, 2 out]
      n94 = call <vilib>:"CTRE_Phoenix_MotorControl_RefNumRegistrySet.vi"("error in (no error)"=w225, "refnum name"="Shooter", "PhoenixMotorControlDevRef"=w224) -> ()  [unwired: 7 in, 2 out]
      n95 = call-poly <vilib>:"SPARK Open.vi"("Invert"=TRUE, "Device Number"=u8 57) -> ("error out"=w63:errorcluster, "MotorControlDeviceRef"=w64:T18)  [unwired: 8 in]
      n96 = call-poly <vilib>:"SPARK Open.vi"("Invert"=FALSE, "Device Number"=u8 58) -> ("error out"=w29:errorcluster, "MotorControlDeviceRef"=w30:T18)  [unwired: 8 in]
      n97 = call-poly <vilib>:"SPARK Configure Closed Loop.vi"("error in"=w63, "Feedback Sensor (Primary Encoder)"=SPARK_Feedback_Sensor."Primary Encoder", "MotorControlDeviceRef in"=w64) -> ("error out"=w74:errorcluster, "MotorControlDeviceRef out"=w76:T18)  [unwired: 7 in]
      n98 = call-poly <vilib>:"SPARK Configure Closed Loop.vi"("error in"=w29, "Feedback Sensor (Primary Encoder)"=SPARK_Feedback_Sensor."Primary Encoder", "MotorControlDeviceRef in"=w30) -> ("error out"=w49:errorcluster, "MotorControlDeviceRef out"=w47:T18)  [unwired: 7 in]
      n99 = call <vilib>:"SPARK Set Sensor Position.vi"("Sensor (Primary Encoder)"=enum16{"Primary Encoder", "Alt/Ext Encoder"}."Primary Encoder", "error in"=w74, "Position"=0.0, "MotorControlDeviceRef"=w76) -> ("error out"=w72:errorcluster, "MotorControlDeviceRef"=w73:T18)  [unwired: 6 in]
      n100 = call <vilib>:"SPARK Set Sensor Position.vi"("Sensor (Primary Encoder)"=enum16{"Primary Encoder", "Alt/Ext Encoder"}."Primary Encoder", "error in"=w49, "Position"=0.0, "MotorControlDeviceRef"=w47) -> ("error out"=w51:errorcluster, "MotorControlDeviceRef"=w50:T18)  [unwired: 6 in]
      n101 = call-poly <vilib>:"SPARK Configure Closed Loop.vi"("error in"=w72, "PID Gains"=T9 {"kP"=0.15, "kI"=0.0, "kD"=0.0}, "MotorControlDeviceRef in"=w73) -> ("error out"=w88:errorcluster, "MotorControlDeviceRef out"=w89:T18)  [unwired: 7 in]
      n102 = call-poly <vilib>:"SPARK Configure Closed Loop.vi"("error in"=w51, "PID Gains"=T9 {"kP"=0.15, "kI"=0.0, "kD"=0.0}, "MotorControlDeviceRef in"=w50) -> ("error out"=w35:errorcluster, "MotorControlDeviceRef out"=w34:T18)  [unwired: 7 in]
      n103 = call-poly <vilib>:"NT Write Value.vi"("value"="Stop" ("default value"), "name"="Climb/Climb Status") -> ()  [unwired: 9 in, 1 out]
      n104 = call-poly <vilib>:"NT Write Value.vi"("value"="Stop" ("default value"), "name"="Climb/Climb Diection") -> ()  [unwired: 9 in, 1 out]
      n105 = call-poly <vilib>:"SPARK Configure Closed Loop.vi"("error in (no error)"=w88, "Compensated Nominal Voltage"=12.0, "Voltage Mode (Disabled)"=Closed_Loop_Voltage_Mode."Voltage Compensation", "MotorControlDeviceRef in"=w89) -> ("error out"=w80:errorcluster, "MotorControlDeviceRef out"=w81:T18)  [unwired: 6 in]
      n106 = call-poly <vilib>:"SPARK Configure Closed Loop.vi"("error in (no error)"=w35, "Compensated Nominal Voltage"=12.0, "Voltage Mode (Disabled)"=Closed_Loop_Voltage_Mode."Voltage Compensation", "MotorControlDeviceRef in"=w34) -> ("error out"=w43:errorcluster, "MotorControlDeviceRef out"=w42:T18)  [unwired: 6 in]
      n107 = call-poly <vilib>:"SPARK Configure Closed Loop.vi"("error in (no error)"=w80, "MotorControlDeviceRef in"=w81) -> ("error out"=w78:errorcluster, "MotorControlDeviceRef out"=w79:T18)  [unwired: 8 in]
      n108 = call-poly <vilib>:"SPARK Configure Closed Loop.vi"("error in (no error)"=w43, "MotorControlDeviceRef in"=w42) -> ("error out"=w45:errorcluster, "MotorControlDeviceRef out"=w44:T18)  [unwired: 8 in]
      n109 = call-poly <vilib>:"SPARK Configure Basic.vi"("error in (no error)"=w78, "Idle Mode"=Spark_MAX_Idle_Mode."Brake", "MotorControlDeviceRef in"=w79) -> ("error out"=w82:errorcluster, "MotorControlDeviceRef out"=w83:T18)  [unwired: 7 in]
      n110 = call-poly <vilib>:"SPARK Configure Basic.vi"("error in (no error)"=w45, "Idle Mode"=Spark_MAX_Idle_Mode."Brake", "MotorControlDeviceRef in"=w44) -> ("error out"=w41:errorcluster, "MotorControlDeviceRef out"=w40:T18)  [unwired: 7 in]
      n111 = Divide(x=w301, y=2.0) -> (x/y=w299:dbl)
      n112 = Divide(x=w292, y=2.0) -> (x/y=w294:dbl)
      n113 = Reciprocal(x=w299) -> (1/x=w298:dbl)
      n114 = call-poly <vilib>:"SPARK Configure Power.vi"("error in (no error)"=w82, "Primay Current Limit (80A)"=40.0, "MotorControlDeviceRef in"=w83) -> ("error out"=w85:errorcluster, "MotorControlDeviceRef out"=w86:T18)  [unwired: 7 in]
      n115 = call-poly <vilib>:"SPARK Configure Power.vi"("error in (no error)"=w41, "Primay Current Limit (80A)"=40.0, "MotorControlDeviceRef in"=w40) -> ("error out"=w38:errorcluster, "MotorControlDeviceRef out"=w37:T18)  [unwired: 7 in]
      n116 = Reciprocal(x=w294) -> (1/x=w295:dbl)
      n117 = Compound Arithmetic op=MULTIPLY(w297, w298, w119) -> (w25:dbl)
      n118 = Compound Arithmetic op=MULTIPLY(w296, w295, w125) -> (w59:dbl)
      n119 = call-poly <vilib>:"SPARK Configure Encoder.vi"("error in"=w85, "MotorControlDeviceRef in"=w86) -> ("error out"=w65:errorcluster, "MotorControlDeviceRef out"=w66:T18)  [unwired: 8 in]
      n120 = call-poly <vilib>:"SPARK Configure Encoder.vi"("error in"=w38, "MotorControlDeviceRef in"=w37) -> ("error out"=w58:errorcluster, "MotorControlDeviceRef out"=w57:T18)  [unwired: 8 in]
      n121 = Divide(x=w120, y=2.0) -> (x/y=w122:dbl)
      n122 = call-poly <vilib>:"SPARK Configure Soft Limit.vi"("error in"=w65, "Enabled? (T)"=FALSE, "Soft Limit"=w59, "MotorControlDeviceRef in"=w66) -> ("error out"=w67:errorcluster, "MotorControlDeviceRef out"=w68:T18)  [unwired: 6 in]
      n123 = call-poly <vilib>:"SPARK Configure Soft Limit.vi"("error in"=w58, "Enabled? (T)"=FALSE, "Soft Limit"=w25, "MotorControlDeviceRef in"=w57) -> ("error out"=w56:errorcluster, "MotorControlDeviceRef out"=w55:T18)  [unwired: 6 in]
      n124 = Divide(x=w130, y=2.0) -> (x/y=w128:dbl)
      n125 = Reciprocal(x=w122) -> (1/x=w123:dbl)
      n126 = Reciprocal(x=w128) -> (1/x=w127:dbl)
      n127 = Compound Arithmetic op=MULTIPLY(w124, w123, w119) -> (w26:dbl)
      n128 = Compound Arithmetic op=MULTIPLY(w126, w127, w125) -> (w60:dbl)
      n129 = call-poly <vilib>:"SPARK Configure Soft Limit.vi"("error in"=w67, "Enabled? (T)"=FALSE, "Soft Limit"=w60, "MotorControlDeviceRef in"=w68) -> ("error out"=w61:errorcluster, "MotorControlDeviceRef out"=w62:T18)  [unwired: 6 in]
      n130 = call-poly <vilib>:"SPARK Configure Soft Limit.vi"("error in"=w56, "Enabled? (T)"=FALSE, "Soft Limit"=w26, "MotorControlDeviceRef in"=w55) -> ("error out"=w27:errorcluster, "MotorControlDeviceRef out"=w28:T18)  [unwired: 6 in]
      n131 = call <vilib>:"WPI_MotorControlRefNum Registry Set.vi"("error in (no error)"=w27, "refnum name"="Climb R", "MotorControlDevRef"=w28) -> ()  [unwired: 7 in, 2 out]
      n132 = call <vilib>:"WPI_MotorControlRefNum Registry Set.vi"("error in (no error)"=w61, "refnum name"="Climb L", "MotorControlDevRef"=w62) -> ()  [unwired: 7 in, 2 out]
      n133 = call-poly <vilib>:"NT Write Value.vi"("value"=w125, "name"="Climb/Gear Ratio/Climb L") -> ()  [unwired: 9 in, 1 out]
      n134 = call-poly <vilib>:"NT Write Value.vi"("value"=w119, "name"="Climb/Gear Ratio/Climb R") -> ()  [unwired: 9 in, 1 out]
    }
    frame Enabled {
    }
  }
  "error out" <- "error in"
